vi "Configure Sequence ARB TDD Mode.vi"(8 "error in (no error)":errorcluster, 9 "TDD Mode (Off)":bool, 10 "Instance (1)":i32=1, 11 "VISA resource name":refnum<visa-resource-name>) -> (0 "error out":errorcluster, 3 "VISA resource name out":refnum<visa-resource-name>)   [LabVIEW 2020, in "Rohde&Schwarz CMXP GPRF.lvlib"]
doc: "Enables or disables the TDD mode for a signal output path with a remote radio head (RRH).\n\nAttribute(s):\nRSCMXPGPRF_ATTR_SEQUENCER_ARB_TDD_MODE\n\nRemote-control command(s):\nSOURce:GPRF:GEN<i>:SEQuencer:NREPetition"
uses:
  <instrlib>/Rohde&Schwarz CMXP GPRF/Rohde&Schwarz CMXP GPRF.lvlib
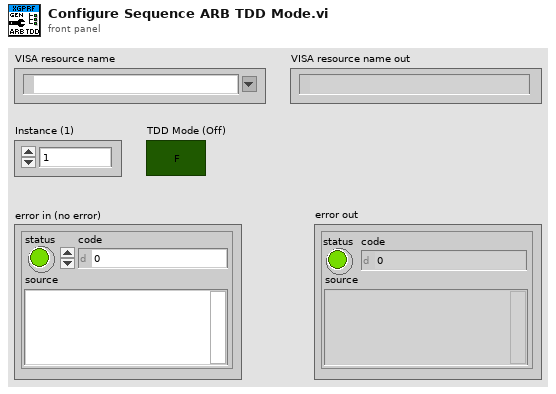
[diagram p1: front panel]
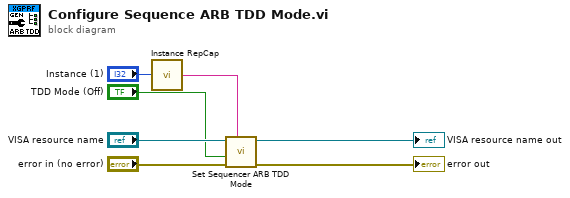
[diagram p0: block diagram]
diagram:
  n1 = call <instrlib>:"Instance RepCap.vi"("Instance in"="Instance (1)") -> ("Instance out"=w3:string)
  n2 = call "Set Sequencer ARB TDD Mode"("Repeated Capabilities"=w3, "error in (no error)"="error in (no error)", "Sequencer ARB TDD Mode (OFF)"="TDD Mode (Off)", "instrument handle"="VISA resource name") -> ("error out"=→"error out":errorcluster, "instrument handle out"=→"VISA resource name out":refnum<visa-resource-name>)  [unwired: 6 in]
